vi "GEA2 Serial ICP Dryer SM.vi"(0 "ComPort":refnum<visa-resource-name>="COM1", 5 "Mode":T6=enum."Send WILT Startup CMDs", 7 "Xtra Command Data":u8[](array[numeric]) format="%02x", 9 "Dryer Status Serial Data In":T2, 11 "Error In":errorcluster, 13 "Command":T5 items=["CMD_Eval_Mode_Entry_CC1", "CMD_Eval_Mode_Entry_CC2", "CMD_Eval_Mode_Continue", "CMD_Send_DIAG_Info", "CMD_Enable_Debug_Log ", "CMD_Disable_Debug_Log ", "CMD_Send_Log_Data", "CMD_Stop", "RQST_Version"]) -> (4 "Dryer Status Serial Data Out":T2={"Color"=0, "Last Read Status"=enum."Err", "Command:Data"="", "Com Port"=0, "Time(S)"=0.0, "Err Count"=0}, 8 "DataReturned":u8[](array[numeric]) format="%.0x", 10 "WriteOK":bool, 14 "CRC Match":bool, 15 "Error Out":errorcluster)   [LabVIEW 2014]
uses:
  Type Definitions/GEA2 Serial Dryer Interface Ctrl.ctl
  Type Definitions/GEA2 Serial Dryer Commands.ctl
  Dryer Wilt/Type Definitions/WILT Dryer Com Port Info.ctl
  Dryer Wilt/Type Definitions/WILT Dryer Status Ctrl.ctl
  Type Definitions/Source Destination Control.ctl
  Type Definitions/GEA2 Serial Dryer Error Enumeration.ctl
  GEA2 Serial Globals Dryer.vi
  <vilib>/Instr/_visa.llb/VISA Configure Serial Port (Instr).vi
panel:
  in  "Source Destination 2":T1 {"Destination" format="%x"; "Source" format="%x"}
  in  "Source Destination":T1 {"Destination" format="%x"; "Source" format="%x"}
  in  "Total Bytes Read":i32
  in  "Tab Control 2":enum32{"Debug", "Serial Setup"}(tab)
  in  "Debug":bool
  out "State Array":string[](array[string])
  in  "Serial Timeout":u32=10
  out "Com:Data Buffer":string
  in  "Tab Control":T4(tab)
  in  "Exit":bool
  out "Com:Data":string
  out "Length":u8
  out "Source Read":u8 format="%.0x"
  out "Destination Read":u8 format="%.0x"
  out "Bytes At Port":u32=40
  out "Num Messages":dbl
  out "Read Pulse":dbl
  out "Partial Message":bool
  # "SubVI Commands"
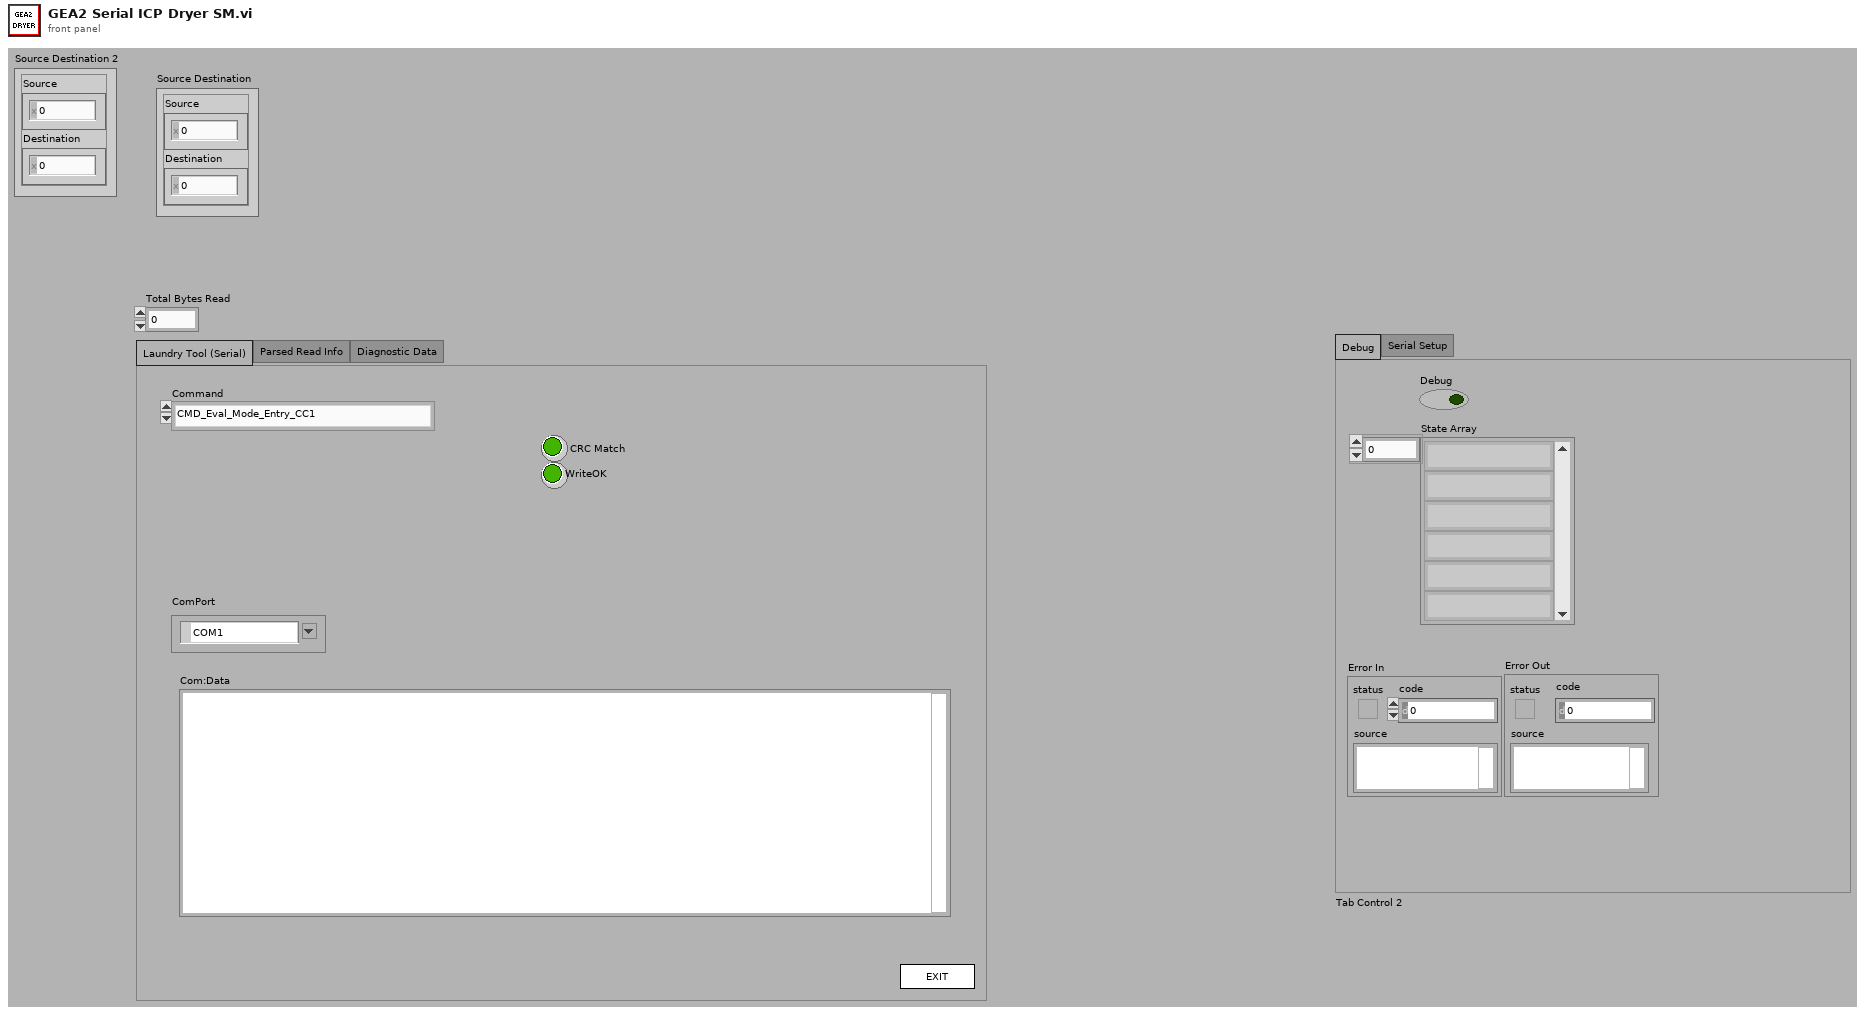
[diagram p1: front panel]
types:
  T1 = typedef "Source Destination Control.ctl" = cluster{"Source":u8, "Destination":u8}
  T2 = typedef "WILT Dryer Com Port Info.ctl" = cluster{"Color":u32, "Last Read Status":T3, "Command:Data":string, "Com Port":u8, "Time(S)":dbl, "Err Count":u32}
  T3 = typedef "WILT Dryer Status Ctrl.ctl" = enum16{"Cycle Not Started", "Cycle Running", "Paused", "Cycle Completed", "Eval Mode Entered", "Err", "Pause (No GEA2)"}
  T4 = enum32{"Laundry Tool (Serial)", "Parsed Read Info", "Diagnostic Data"}
  T5 = typedef "GEA2 Serial Dryer Commands.ctl" = u8
  T6 = typedef "GEA2 Serial Dryer Interface Ctrl.ctl" = enum16{"Init Com Port", "SendCMD", "ReadPort", "Close Port", "Simulate Diag Data", "Send WILT Startup CMDs", "Send Continue CMD", "Read Continuous"}
  T7 = enum32{"invalid app kind", "Development System", "Run Time System", "Student Edition", "Embedded LabVIEW", "Evaluation", "Custom"}
  T8 = enum32{"Invalid", "Standard", "Closed", "Hidden", "Minimized", "Maximized"}
  T9 = typedef "GEA2 Serial Dryer Error Enumeration.ctl" = enum16{"No Error", "GEA2 Send ACK Mismatch", "GEA2 STX", "GEA2 ETX", "GEA2 CRC Mismatch", "GEA2 ReadACK", "RTD In Range Error", "Fail Mean Tank Temp", "No Flow Config Data Found", "Failed Flow During Purge", "Temp During Purge", "Confirm IF Stop Fail", "Init Draw: TC_1 Out of Range", "Flow = 0 During Draw after 20s"}
  T10 = cluster{"Core":cluster{"Current VI Reference":refnum<vi>, "Close Panel on Exit?":bool}, "ComPort":refnum<visa-resource-name>, "ReadArray":u8[], "CRCArray":u8[], "Bytes Remaining":u8, "CRCRead":u8[], "CRC":bool, "Dryer Command":T5, "Error Out Flag":bool, "Bytes Data":u8[], "Dryer Status Serial Data In":T2, "Current Read Index":i32, "Total Bytes Read":i32, "Reset MSG Count":bool, "ACK":bool, "ReadCM1Flag":bool, "ReadCM2Flag":bool, "Reset Pulse":bool}
  T11 = cluster{"Current VI Reference":refnum<vi>, "Close Panel on Exit?":bool}
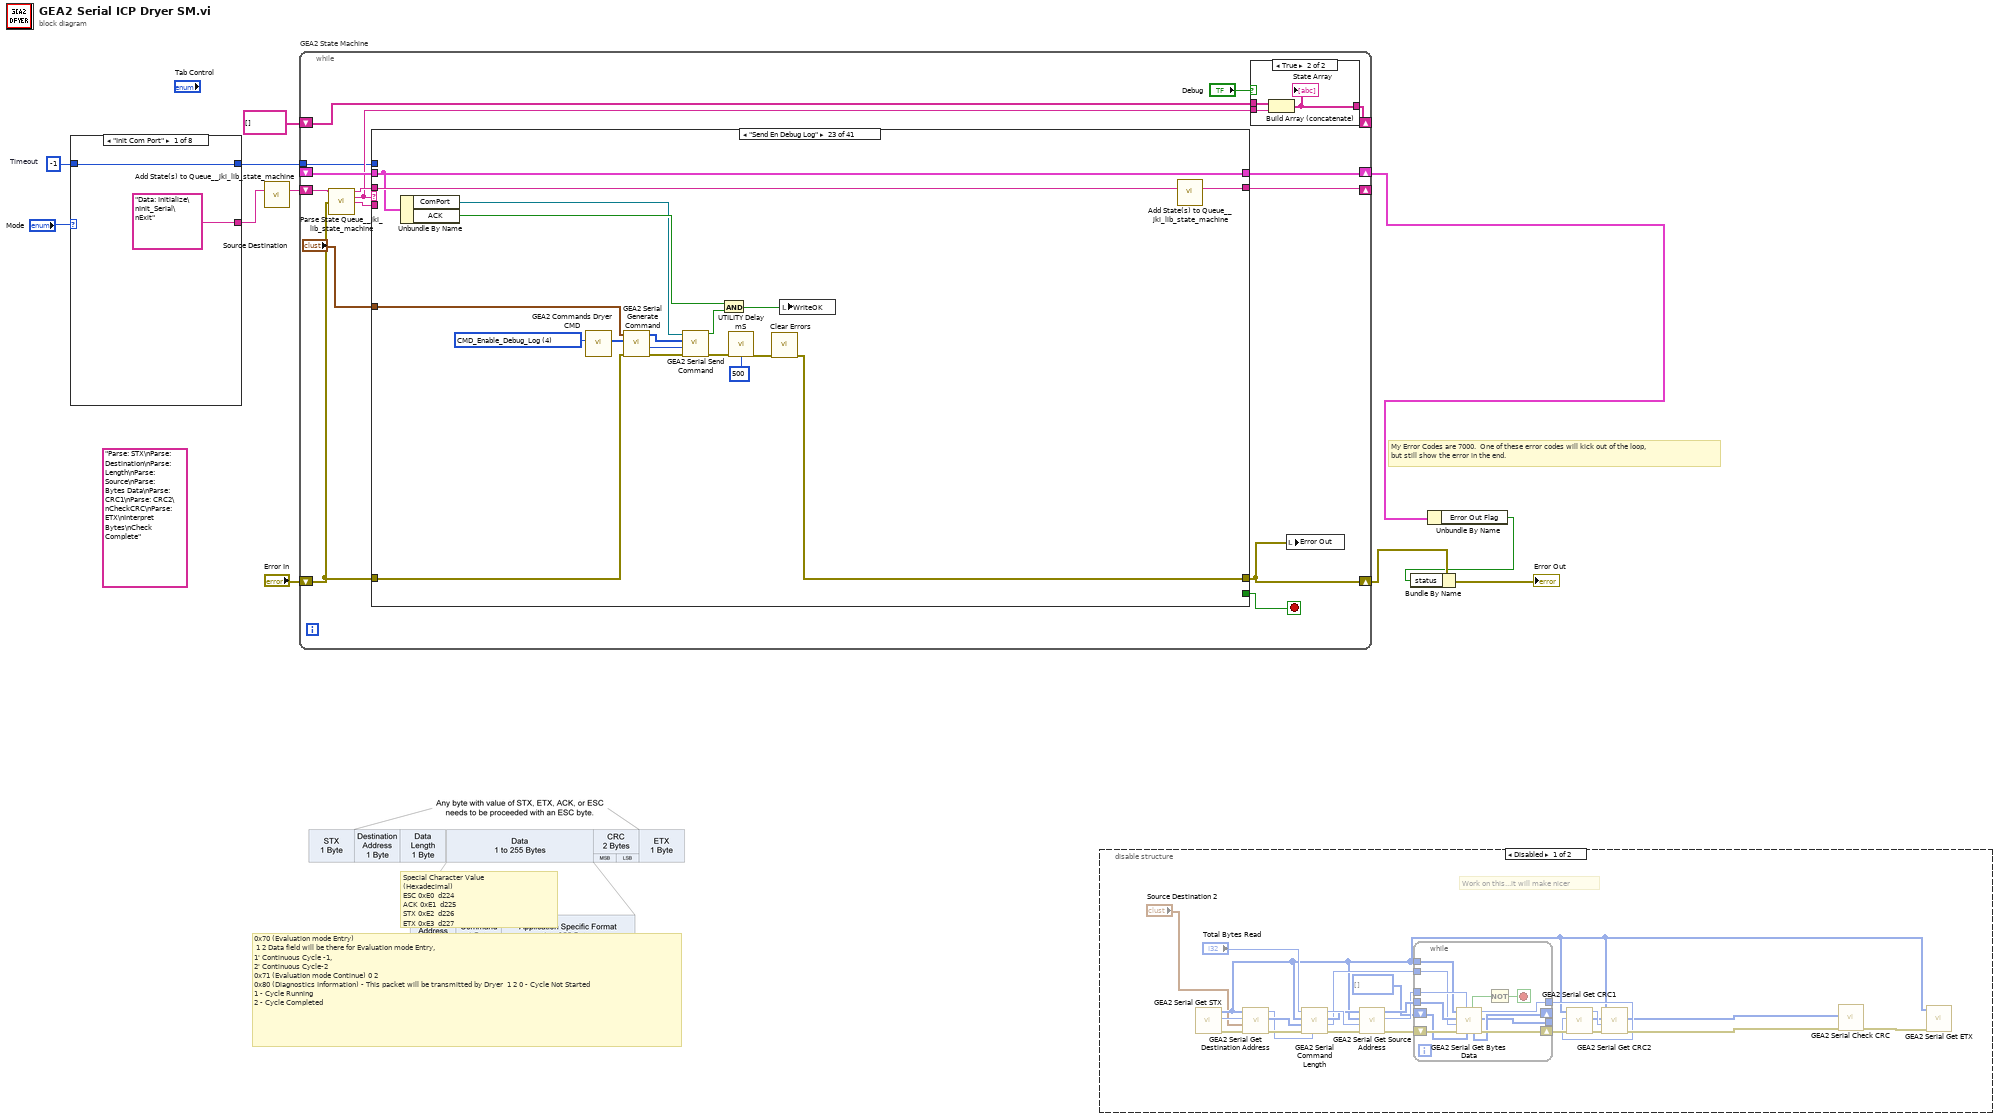
[diagram p0: block diagram]
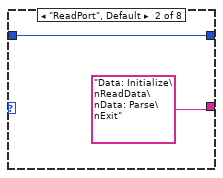
[diagram p3: hidden frame]
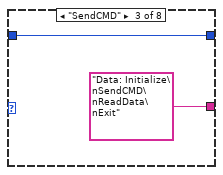
[diagram p4: hidden frame]
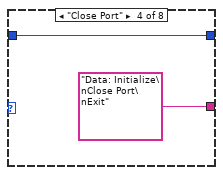
[diagram p5: hidden frame]
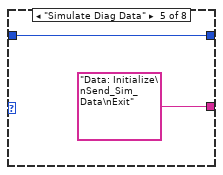
[diagram p6: hidden frame]
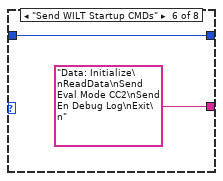
[diagram p7: hidden frame]
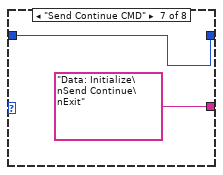
[diagram p8: hidden frame]
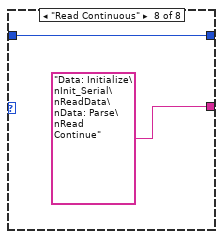
[diagram p9: hidden frame]
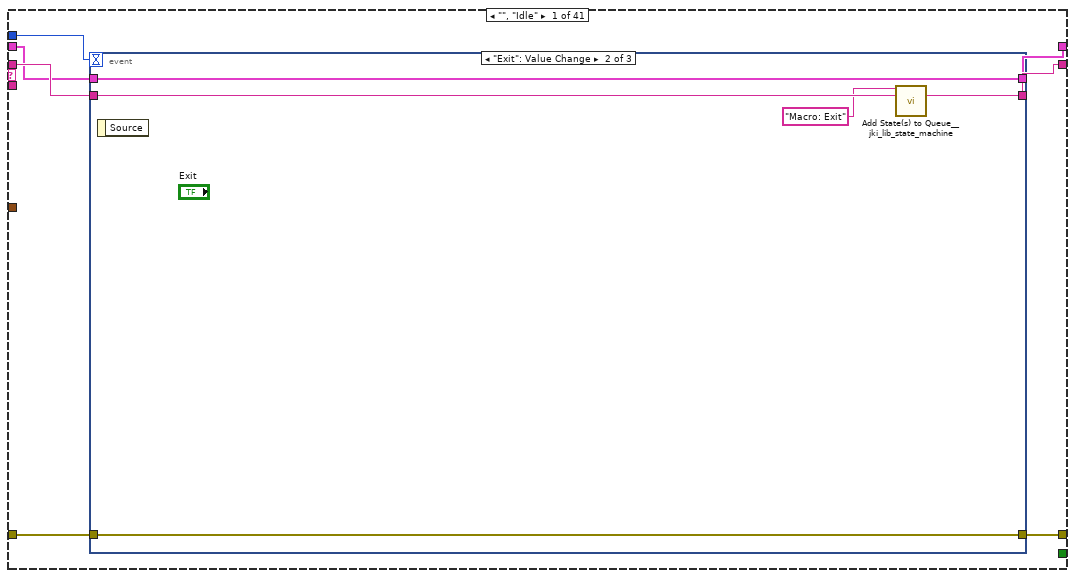
[diagram p11: hidden frame]
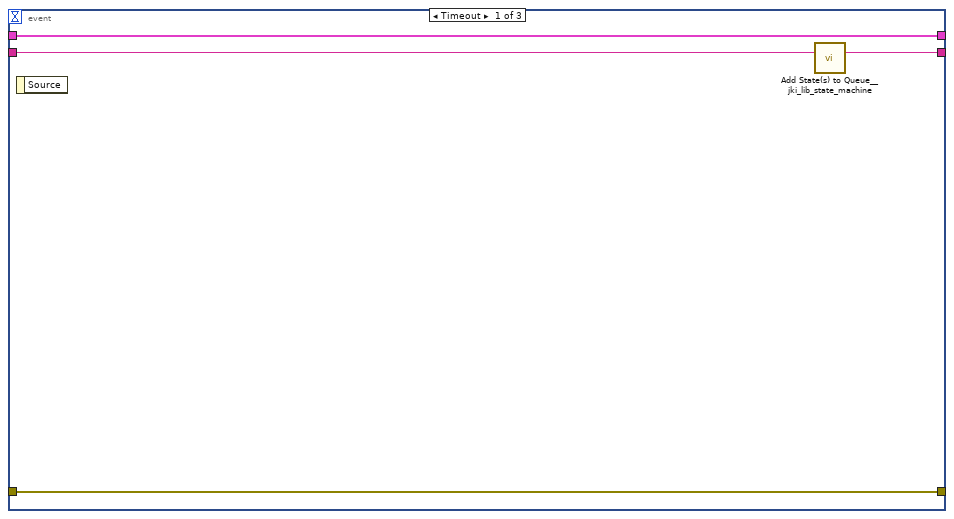
[diagram p12: hidden frame]
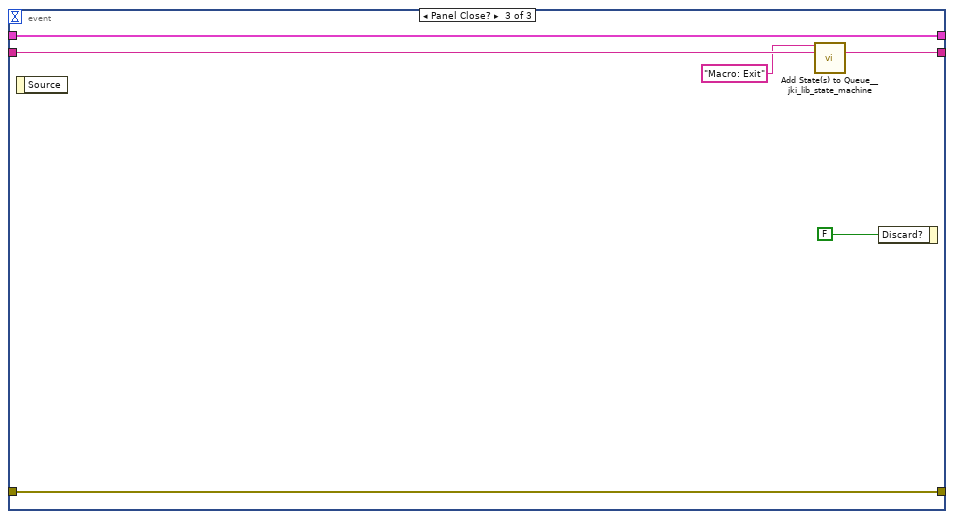
[diagram p13: hidden frame]
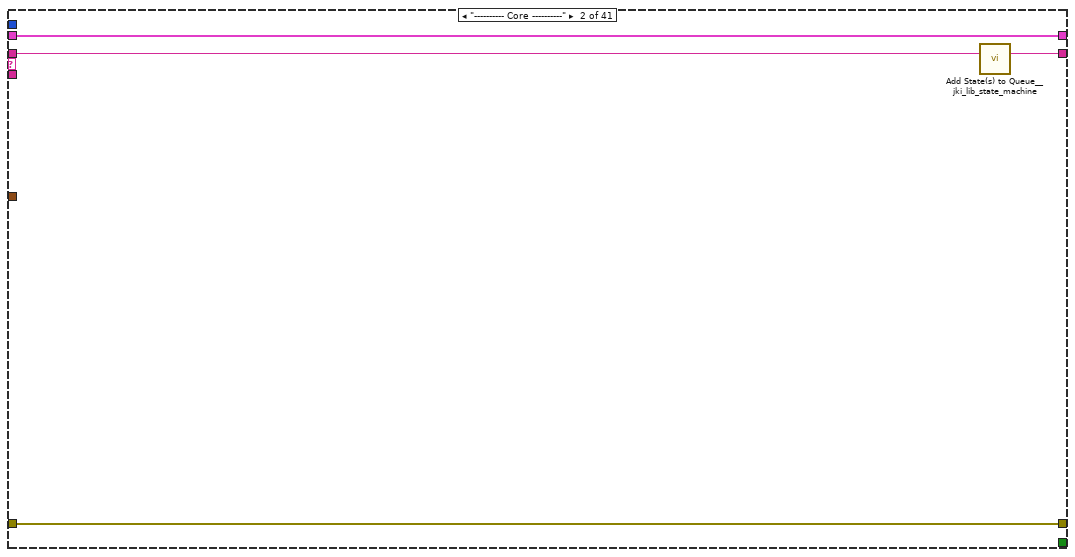
[diagram p14: hidden frame]
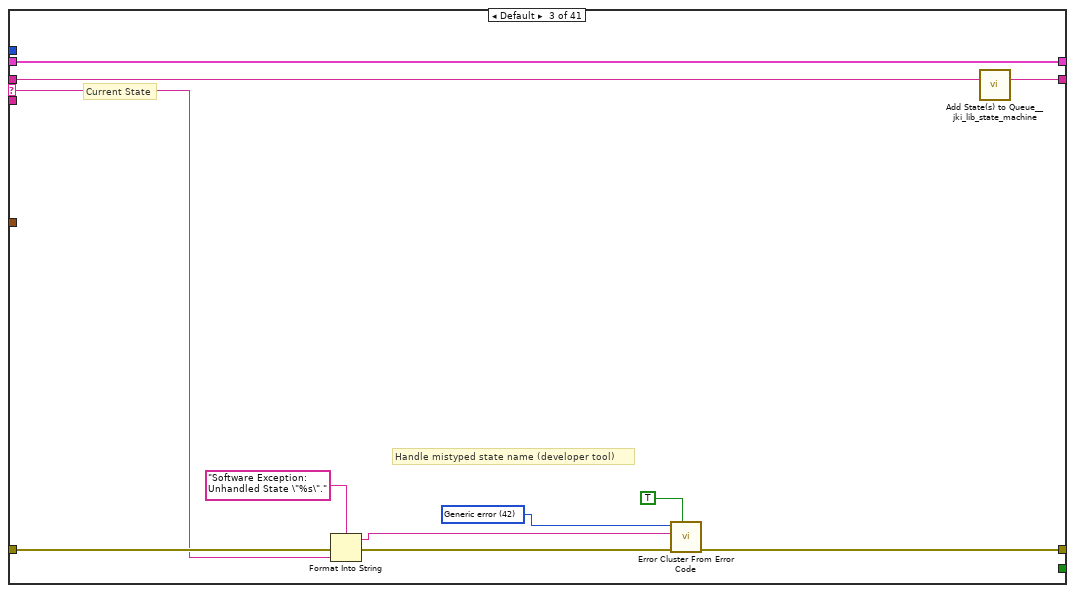
[diagram p15: hidden frame]
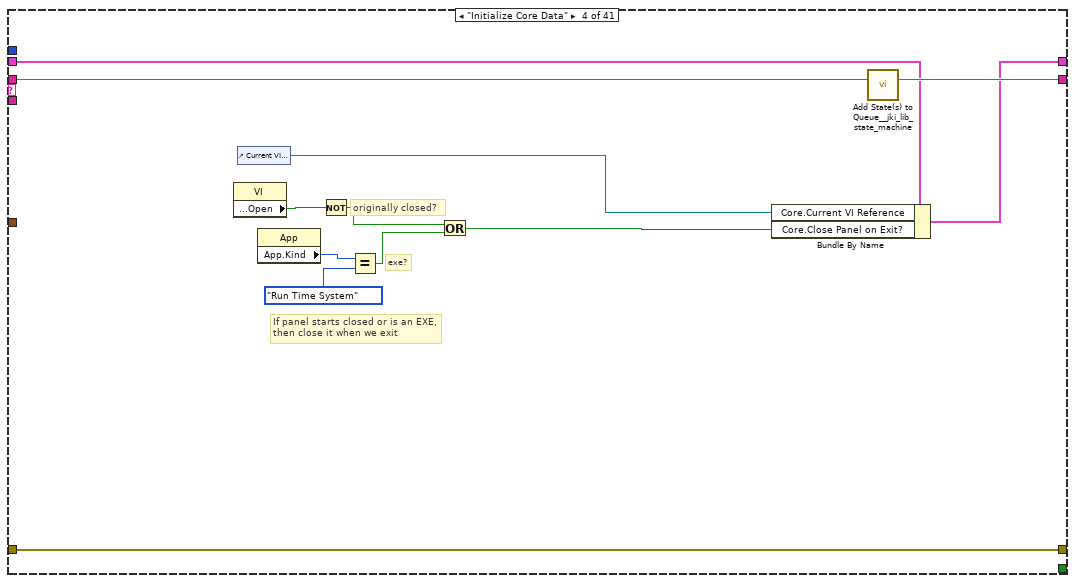
[diagram p16: hidden frame]
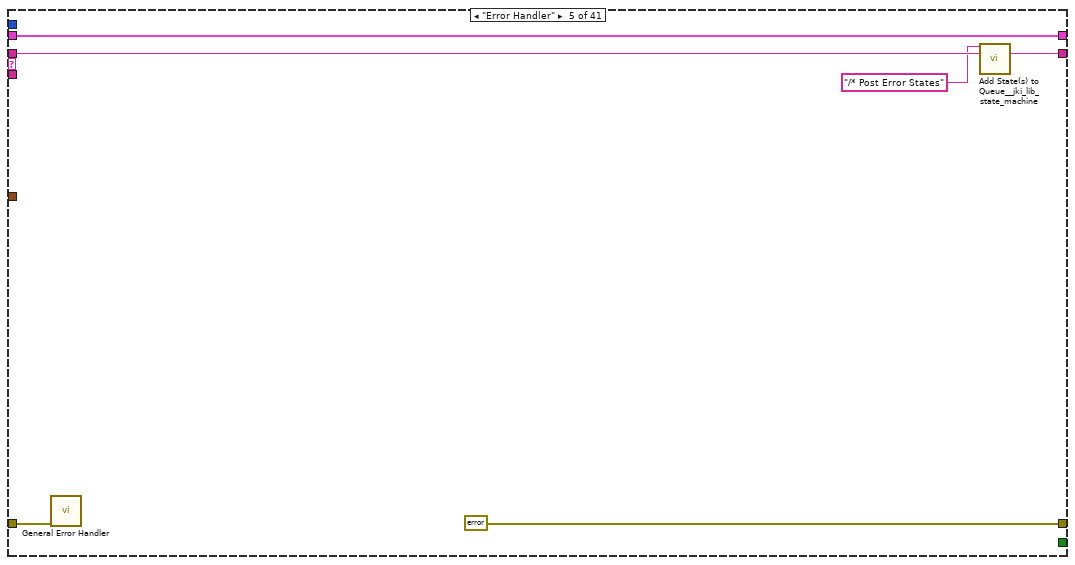
[diagram p17: hidden frame]
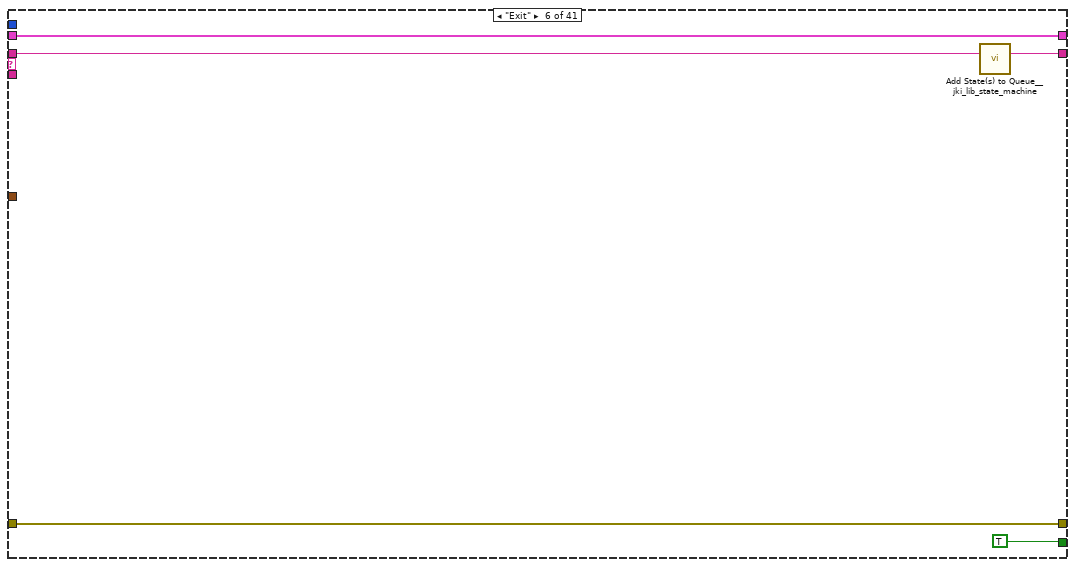
[diagram p18: hidden frame]
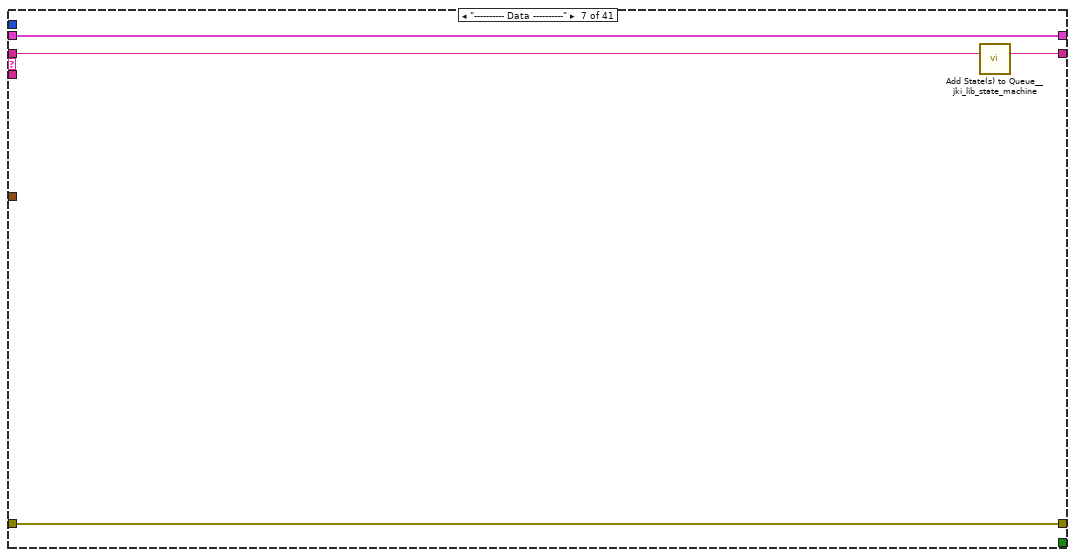
[diagram p19: hidden frame]
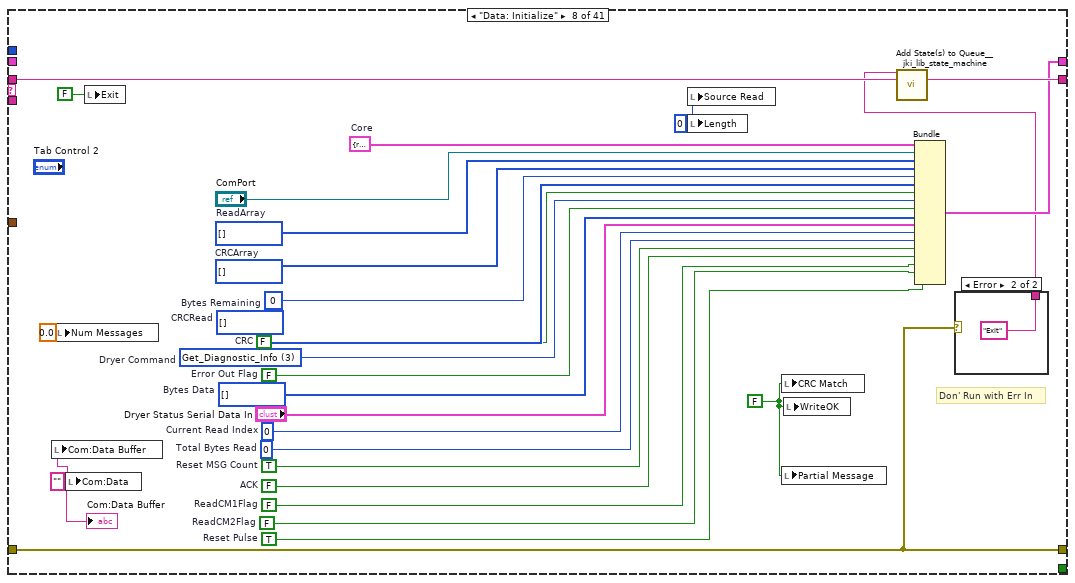
[diagram p20: hidden frame]
diagram:
  (unwired) "Parse: STX\nParse: Destination\nParse: Length\nParse: Source\nParse: Bytes Data\nParse: CRC1\nParse: CRC2\nCheckCRC\nParse: ETX\nInterpret Bytes\nCheck Complete" ("State(s) in Front (\"\")")
  w2 = -1  # Timeout
  # "0x70 (Evaluation mode Entry) \n\t1\t2\tData field will be there for Evaluation mode Entry, \n1' Continuous Cycle -1, \n2' Continuous Cycle-2\n0x71 (Evaluation mode Continue)\t0\t2\t\n0x80 (Diagnostics Information) - This packet will be transmitted by Dryer \t1\t2\t0 - Cycle Not Started\n1 - Cycle Running\n2 - Cycle Completed"
  # "My Error Codes are 7000.  One of these error codes will kick out of the loop,\nbut still show the error in the end."
  # "Special Character\tValue (Hexadecimal)\nESC\t0xE0  d224\nACK\t0xE1  d225\nSTX\t0xE2  d226\nETX\t0xE3  d227"
  n1 = case shown="\"Init Com Port\"" "Mode" {
    tunnel: ["Data: Initialize\nInit_Serial\nExit" "Data: Initialize\nReadData\nData: Parse\nExit" "Data: Initialize\nSendCMD\nReadData\nExit" "Data: Initialize\nClose Port\nExit" "Data: Initialize\nSend_Sim_Data\nExit" "Data: Initialize\nReadData\nSend Eval Mode CC2\nSend En Debug Log\nExit\n" "Data: Initialize\nSend Continue\nExit" "Data: Initialize\nInit_Serial\nReadData\nData: Parse\nRead Continue"] -> w1
    tunnel: [w12 w14 w16 w18 w20 w22 w24 w27] -> w3
    tunnel: w2 -> [w12 w14 w16 w18 w20 w22 w24 w27]
    frame "Init Com Port" {
    }
    frame "ReadPort", Default {
    }
    frame "SendCMD" {
    }
    frame "Close Port" {
    }
    frame "Simulate Diag Data" {
    }
    frame "Send WILT Startup CMDs" {
    }
    frame "Send Continue CMD" {
    }
    frame "Read Continuous" {
    }
  }
  n2 = call <vilib>:"Add State(s) to Queue__jki_lib_state_machine.vi"("State(s) in (\"\")"=w1) -> ("States Out"=w11:string)  [unwired: 14 in]
  n3 = while "GEA2 State Machine" {
    shift-right: [w38] -> w6
    shift-left: _ -> [w37]
    shift-right: [w34] -> w9
    shift-left: "Error In" -> [w36]
    shift-right: [w35] -> _
    shift-left: w11 -> [w40]
    shift-right: [w31] -> _
    shift-left: string[] [] -> [w33]
    tunnel: w3 -> [w30]
    stop <- w39 stop-if-true
    n4 = call <vilib>:"Parse State Queue__jki_lib_state_machine.vi"("State Queue"=w40, "Error In (no error)"=w36) -> ("Remaining States"=w42:string, "Current State"=w32:string, "Arguments"=w41:string)  [unwired: 11 in]
    n5 = case shown="\"Send En Debug Log\"" w32 {
      selector: w32 -> [_ _ w73 _ _ _ _ _ _ _ _ _ _ _ _ _ _ _ _ _ _ _ _ _ _ _ _ _ _ _ _ _ _ _ _ _ _ _ _ _ _]
      tunnel: w42 -> [w53 w72 w77 w95 w101 w102 w110 w138 w145 w149 w153 w159 w170 w196 w201 w211 w215 w241 w252 w270 w287 w302 w320 w334 w346 w363 w367 w376 w396 w415 w423 w449 w466 w478 w489 w498 w510 w524 w534 w548 w574]
      tunnel: w41 -> [_ _ _ _ _ _ _ _ _ _ _ w154 w164 _ _ _ _ _ _ _ _ _ _ _ _ _ _ _ _ _ _ _ _ _ _ _ _ _ _ _ _]
      tunnel: w37 -> [w51 w69 w75 w86 w97 w104 w107 _ w142 w146 w151 w157 w166 w193 w198 w208 w212 w238 w249 w262 w284 w299 w317 w330 w344 w360 w364 w370 w394 w413 w431 w447 w464 w476 w487 w494 w508 w519 w529 w537 w555]
      tunnel: [w50 w70 w79 w92 errorcluster {"status"=FALSE, "code"=0, "source"=""} ("error out") w105 w108 w124 w140 w147 w150 w155 w167 w194 w199 w209 w213 w239 w250 w264 w282 w297 w312 w321 w335 w347 w365 w374 w392 w404 w416 w438 w451 w469 w479 w492 w505 w520 w532 w546 w572] -> w34
      tunnel: w36 -> [w49 w70 w78 w92 w99 w105 w108 w124 w143 w147 w150 w156 w168 w194 w199 w209 w213 w225 w247 w255 w279 w296 w311 w331 w338 w354 w365 w374 w386 w405 w417 w439 w452 w470 w480 w496 w500 w522 w532 w546 w572]
      tunnel: [w52 w71 w76 w94 w100 w106 w109 w137 w144 w148 w152 w158 w169 w195 w200 w210 w214 w240 w251 w269 w286 w301 w319 w333 w345 w362 w366 w375 w395 w414 w432 w448 w465 w477 w488 w497 w509 w523 w533 w547 w573] -> w35
      tunnel: [_ _ _ _ _ TRUE _ _ _ _ _ _ _ _ _ _ _ _ _ _ _ _ _ _ _ _ _ _ _ _ _ _ _ _ _ _ _ _ _ _ _] -> w39
      tunnel: [w48 w69 w75 w93 w97 w104 w107 w136 w142 w146 w151 w157 w166 w193 w198 w208 w212 w237 w249 w262 w283 w299 w317 w330 w344 w356 w364 w369 w393 w412 w430 w446 w463 w475 w486 w493 w507 w519 w528 w536 w571] -> w38
      tunnel: w30 -> [w47 _ _ _ _ _ _ _ _ _ _ _ _ _ _ _ _ _ _ _ _ _ _ _ _ _ _ _ _ _ _ _ _ _ _ _ _ _ _ _ _]
      tunnel: "Source Destination" -> [_ _ _ _ _ _ _ _ _ _ _ _ _ _ _ _ _ _ _ w253 w281 w293 w310 w329 w343 _ _ _ _ _ _ w441 _ _ _ _ _ _ _ _ _]
      frame "", "Idle" {
        n6 = event shown="[1] \"Exit\": Value Change" {
          selector: _ -> [_ _ _]
          dyn-events: _ -> [_ _ _]
          timeout: w47 -> [_ _ _]
          tunnel: w53 -> [w57 w62 w68]
          tunnel: [w56 w61 w67] -> w52
          tunnel: w51 -> [w54 w59 w65]
          tunnel: [w55 w60 w66] -> w50
          tunnel: w49 -> [w55 w60 w66]
          tunnel: [w54 w59 w65] -> w48
          event Timeout {
            n7 = event-data() -> ()  [unwired: 1 in, 1 out]
            n8 = call <vilib>:"Add State(s) to Queue__jki_lib_state_machine.vi"("State(s) in (\"\")"=w57) -> ("States Out"=w56:string)  [unwired: 14 in]
          }
          event "Exit": Value Change {
            n9 = event-data() -> ()  [unwired: 1 in, 1 out]
            n10 = call <vilib>:"Add State(s) to Queue__jki_lib_state_machine.vi"("State(s) in Front (\"\")"="Macro: Exit", "State(s) in (\"\")"=w62) -> ("States Out"=w61:string)  [unwired: 13 in]
          }
          event Panel Close? {
            n11 = event-data() -> ()  [unwired: 1 in, 1 out]
            n12 = call <vilib>:"Add State(s) to Queue__jki_lib_state_machine.vi"("State(s) in Front (\"\")"="Macro: Exit", "State(s) in (\"\")"=w68) -> ("States Out"=w67:string)  [unwired: 13 in]
            n13 = event-data("Discard?"=FALSE) -> ()  [unwired: 1 in, 1 out]
          }
        }
      }
      frame "---------- Core ----------" {
        n14 = call <vilib>:"Add State(s) to Queue__jki_lib_state_machine.vi"("State(s) in (\"\")"=w72) -> ("States Out"=w71:string)  [unwired: 14 in]
      }
      frame Default {
        w82 = 42 items=["No error", "Argument error", "Memory is full", "Out of zone", "End of file", "File already open", "Generic file I/O error", "File not found", "File permission error", "Disk is full", "Duplicate path", "Too many files open", "System feature not enabled", "Resource file not found", "Cannot add resource", "Resource not found", "Image not found", "Image memory error", "Pen does not exist", "Config type invalid", "Config token not found", "Config parse error", "Config memory error", "Bad external code format", "Bad external code offset", "External code not present", "Null window", "Destroy window error", "Null menu", "Print aborted", "Bad print record", "Print driver error", "Windows error during printing", "Memory error during printing", "Print dialog error", "Generic print error", "Invalid device refnum", "Device not found", "Device parameter error", "Device unit error", "Cannot open device", "Device call aborted", "Generic error", "Cancelled by user", "Object ID too low", "Object ID too high", "Object not in heap", "Unknown heap", "Unknown object (invalid DefProc)", "Unknown object (DefProc not in table)", "Message out of range", "Invalid (null) method", "Unknown message", "Manager call not supported", "Bad address", "Network operation in progress", "Network operation timed out", "Connection is busy", "Network attribute not supported", "Network error", "Address in use", "System out of memory", "Connection aborted", "Connection refused", "Not connected", "Already connected", "Connection closed", "Initialization error (interapplication manager)", "Bad occurrence", "Wait on unbound occurrence handler", "Occurrence queue overflow", "Datalog type conflict", "Unused", "Unrecognized type (interapplication manager)", "Memory corrupt", "Failed to make temporary DLL", "Old CIN version", "Drag socket not found", "Failed to load drop-object", "Failed to register OLE object", "Failed to release OLE object", "Format specifier type mismatch", "Unknown format specifier", "Too few format specifiers", "Too many format specifiers", "Scan failed", "Newer CIN version", "Error converting to variant", "Runtime menu error", "Password tampered", "Variant attribute not found", "Incompatible variant data type", "Event data is not available", "Event Store is not present", "Occurrence is not found", "Event Queue is not created", "Event info is not available", "Refnum passed is NULL", "Error retrieving Class GUID", "Error retrieving CoClass GUID", "Error retrieving TypeLib GUID.", "Bad built application magic bytes.", "Specific driver is different from the specific driver associated with the Logical Name.", "There is no session opened to the class driver.", "Max Error", "MAX - Error with config objects", "MAX - Error loading configuration", "MAX - Group not supported"]
        # "Current State"
        # "Handle mistyped state name (developer tool)"
        n15 = Format Into String(format string="Software Exception: Unhandled State \"%s\"." ("message"), error in=w78, w73) -> (resulting string=w81:string, error out=w80:errorcluster)  [unwired: 1 in]
        n16 = call <vilib>:"Error Cluster From Error Code.vi"("show call chain? (False)"=TRUE, "error in (no error)"=w80, "error message (\"\")"=w81, "error code (0)"=w82) -> ("error out"=w79:errorcluster)  [unwired: 5 in]
        n17 = call <vilib>:"Add State(s) to Queue__jki_lib_state_machine.vi"("State(s) in (\"\")"=w77) -> ("States Out"=w76:string)  [unwired: 14 in]
      }
      frame "Initialize Core Data" {
        # "originally closed?"
        # "exe?"
        # "If panel starts closed or is an EXE, then close it when we exit"
        n18 = property class="VI"() -> ("Front Panel.Open"=w91:bool)  [unwired: 2 in, 2 out]
        n19 = control-ref of="Current VI Reference"() -> (w84:refnum<vi>)
        n20 = property class="App"() -> ("App.Kind"=w90:T7)  [unwired: 2 in, 2 out]
        n21 = Not(x=w91) -> (.not. x?=w88:bool)
        n22 = Equal?(x=w90, y=T7."Run Time System" ("Application:Kind")) -> (x = y?=w87:bool)
        n23 = Or(x=w88, y=w87) -> (x .or. y?=w85:bool)
        n24 = Bundle By Name(cluster=w86, "Core.Current VI Reference"=w84, "Core.Close Panel on Exit?"=w85) -> (w93:T10)
        n25 = call <vilib>:"Add State(s) to Queue__jki_lib_state_machine.vi"("State(s) in (\"\")"=w95) -> ("States Out"=w94:string)  [unwired: 14 in]
      }
      frame "Error Handler" {
        n26 = call <vilib>:"General Error Handler.vi"("error in (no error)"=w99) -> ()  [unwired: 10 in, 5 out]
        n27 = call <vilib>:"Add State(s) to Queue__jki_lib_state_machine.vi"("State(s) in Front (\"\")"="/* Post Error States", "State(s) in (\"\")"=w101) -> ("States Out"=w100:string)  [unwired: 13 in]
      }
      frame "Exit" {
        n28 = call <vilib>:"Add State(s) to Queue__jki_lib_state_machine.vi"("State(s) in (\"\")"=w102) -> ("States Out"=w106:string)  [unwired: 14 in]
      }
      frame "---------- Data ----------" {
        n29 = call <vilib>:"Add State(s) to Queue__jki_lib_state_machine.vi"("State(s) in (\"\")"=w110) -> ("States Out"=w109:string)  [unwired: 14 in]
      }
      frame "Data: Initialize" {
        w112 = TRUE  # Reset Pulse
        w115 = FALSE  # ReadCM2Flag
        w116 = FALSE  # ReadCM1Flag
        w113 = "" ("Com:Data")
        w117 = FALSE  # ACK
        w118 = TRUE  # Reset MSG Count
        w119 = 0  # Total Bytes Read
        w120 = 0  # Current Read Index
        w125 = u8 0 ("Length")
        w126 = T5 3 items=["Eval_Mode_Entry_CC1", "Eval_Mode_Entry_CC2", "Eval_Mode_Continue", "Get_Diagnostic_Info"]  # Dryer Command
        w127 = u8[] []  # Bytes Data
        w128 = T11 {"Current VI Reference"=refnum, "Close Panel on Exit?"=FALSE}  # Core
        w114 = FALSE ("CRC Match")
        w129 = FALSE  # Error Out Flag
        w130 = FALSE  # CRC
        w131 = u8[] []  # CRCRead
        w132 = u8 0  # Bytes Remaining
        w133 = u8[] []  # CRCArray
        w134 = u8[] []  # ReadArray
        # "Don' Run with Err In"
        n30 = local write "Com:Data Buffer"(w113) -> ()
        n31 = local write "Num Messages"(0.0 ("Num Messages")) -> ()
        n32 = local write "Com:Data"(w113) -> ()
        n33 = local write "Exit"(FALSE ("Start Pressed")) -> ()
        n34 = local write "Source Read"(w125) -> ()
        n35 = local write "Length"(w125) -> ()
        n36 = local write "CRC Match"(w114) -> ()
        n37 = local write "Partial Message"(w114) -> ()
        n38 = local write "WriteOK"(w114) -> ()
        n39 = Bundle("Core"=w128, "ComPort"="ComPort", "ReadArray"=w134, "CRCArray"=w133, "Bytes Remaining"=w132, "CRCRead"=w131, "CRC"=w130, "Dryer Command"=w126, "Error Out Flag"=w129, "Bytes Data"=w127, "Dryer Status Serial Data In"="Dryer Status Serial Data In", "Current Read Index"=w120, "Total Bytes Read"=w119, "Reset MSG Count"=w118, "ACK"=w117, "ReadCM1Flag"=w116, "ReadCM2Flag"=w115, "Reset Pulse"=w112) -> (w136:T10)  [unwired: 1 in]
        n40 = case shown="Error" w124 {
          tunnel: [_ "Exit"] -> w123
          frame No Error {
          }
          frame Error {
          }
        }
        n41 = call <vilib>:"Add State(s) to Queue__jki_lib_state_machine.vi"("State(s) in Front (\"\")"=w123, "State(s) in (\"\")"=w138) -> ("States Out"=w137:string)  [unwired: 13 in]
        "Com:Data Buffer" <- w113
      }
      frame "Data: Cleanup" {
        n42 = Unbundle By Name(w142) -> ("Core.Current VI Reference"=w141:refnum<vi>)
        n43 = Close Reference(reference=w141, error in (no error)=w143) -> (error out=w140:errorcluster)
        n44 = call <vilib>:"Add State(s) to Queue__jki_lib_state_machine.vi"("State(s) in (\"\")"=w145) -> ("States Out"=w144:string)  [unwired: 14 in]
      }
      frame "---------- UI ----------" {
        n45 = call <vilib>:"Add State(s) to Queue__jki_lib_state_machine.vi"("State(s) in (\"\")"=w149) -> ("States Out"=w148:string)  [unwired: 14 in]
      }
      frame "UI: Initialize" {
        n46 = call <vilib>:"Add State(s) to Queue__jki_lib_state_machine.vi"("State(s) in (\"\")"=w153) -> ("States Out"=w152:string)  [unwired: 14 in]
      }
      frame "UI: Cursor Set" {
        # "Argument"
        n47 = case shown="\"Idle\", Default" w154 {
          tunnel: w156 -> [w161 w163]
          tunnel: [w160 w162] -> w155
          frame "Idle", Default {
            n48 = call <vilib>:"Unset Busy.vi"("error in (no error)"=w161) -> ("error out"=w160:errorcluster)  [unwired: 10 in]
          }
          frame "Busy" {
            n49 = call <vilib>:"Set Busy.vi"("error in (no error)"=w163) -> ("error out"=w162:errorcluster)  [unwired: 9 in, 1 out]
          }
        }
        n50 = call <vilib>:"Add State(s) to Queue__jki_lib_state_machine.vi"("State(s) in (\"\")"=w159) -> ("States Out"=w158:string)  [unwired: 14 in]
      }
      frame "UI: Front Panel State" {
        # "Argument"
        n51 = Unbundle By Name(w166) -> ("Core.Current VI Reference"=w165:refnum<vi>)
        n52 = case shown="\"Close\"" w164 {
          tunnel: w168 -> [w174 w187]
          tunnel: [w176 w188] -> w167
          tunnel: w165 -> [w175 w185]
          frame "Open", Default {
            n53 = property class="VI"(reference=w175, error in=w174) -> (reference out=w172:refnum<vi>, error out=w173:errorcluster, "Front Panel.Open"=w171:bool)
            n54 = case shown="False" w171 {
              tunnel: [w179 w182] -> w176
              tunnel: w173 -> [w178 w182]
              tunnel: w172 -> [w177 _]
              frame False {
                n55 = invoke class="VI" method="FP.Open"(reference=w177, error in=w178, "Activate"=TRUE, "State"=T8."Standard") -> (error out=w179:errorcluster)  [unwired: 1 in, 4 out]
              }
              frame True {
              }
            }
          }
          frame "Close" {
            n56 = property class="VI"(reference=w185, error in=w187) -> (reference out=w184:refnum<vi>, error out=w186:errorcluster, "Front Panel.Open"=w183:bool)
            n57 = case shown="True" w183 {
              tunnel: [w189 w192] -> w188
              tunnel: w186 -> [w189 w191]
              tunnel: w184 -> [_ w190]
              frame False {
              }
              frame True {
                n58 = invoke class="VI" method="FP.Close"(reference=w190, error in=w191) -> (error out=w192:errorcluster)  [unwired: 1 in, 2 out]
              }
            }
          }
        }
        n59 = call <vilib>:"Add State(s) to Queue__jki_lib_state_machine.vi"("State(s) in (\"\")"=w170) -> ("States Out"=w169:string)  [unwired: 14 in]
      }
      frame "---------- Macro ----------" {
        n60 = call <vilib>:"Add State(s) to Queue__jki_lib_state_machine.vi"("State(s) in (\"\")"=w196) -> ("States Out"=w195:string)  [unwired: 14 in]
      }
      frame "Macro: Initialize" {
        w197 = "Data: Initialize\nInitialize Core Data\nUI: Initialize\nUI: Front Panel State >> Open\nInit_Serial"  # Data: Initialize Initialize Core Data UI: Initialize UI: Front Panel State >> Open Init_Serial
        n61 = call <vilib>:"Add State(s) to Queue__jki_lib_state_machine.vi"("State(s) in Front (\"\")"=w197, "State(s) in (\"\")"=w201) -> ("States Out"=w200:string)  [unwired: 13 in]
      }
      frame "Macro: Exit" {
        n62 = Unbundle By Name(w208) -> ("Core.Close Panel on Exit?"=w202:bool)
        n63 = Select(t="UI: Front Panel State >> Close", s=w202, f="") -> (s? t:f=w204:string)
        n64 = call <vilib>:"Add State(s) to Queue__jki_lib_state_machine.vi"("State(s) in (\"\")"=w204, "State(s) at Back (\"\")"="Data: Cleanup\nExit") -> ("States Out"=w207:string)  [unwired: 13 in]
        n65 = call <vilib>:"Add State(s) to Queue__jki_lib_state_machine.vi"("State(s) in Front (\"\")"=w207, "State(s) in (\"\")"=w211) -> ("States Out"=w210:string)  [unwired: 13 in]
      }
      frame "---------- New Category ----------" {
        n66 = call <vilib>:"Add State(s) to Queue__jki_lib_state_machine.vi"("State(s) in (\"\")"=w215) -> ("States Out"=w214:string)  [unwired: 14 in]
      }
      frame "Init_Serial" {
        w232 = u16 0 items=["None", "XON/XOFF", "RTS/CTS", "XON/XOFF & RTS/CTS", "DTR/DSR", "XON/XOFF & DTR/DSR"] ("flow control (0:none)")
        w231 = u16 10 items=["1.0"=10, "1.5"=15, "2.0"=20] ("stop bits (10: 1 bit)")
        # "skip error handle routine"
        # "Assumes that if the serial port is 19200, then it is all ok."
        n67 = Unbundle By Name(w238) -> ("ComPort"=w219:refnum<visa-resource-name>)
        n68 = call "UTILITY Com Chan Type Conversion.vi"("Com Chan In"=w219) -> ("Com Channel #"=w218:u8)  [unwired: 11 in, 3 out]
        n69 = global read "GEA2 Serial Globals Dryer.vi" "No Com Color"() -> (w224:u32)
        n70 = Bundle By Name(cluster=T2 {"Color"=0, "Last Read Status"=enum."Err", "Command:Data"="", "Com Port"=0, "Time(S)"=0.0, "Err Count"=0} ("Dryer Status Serial Data Out"), "Color"=w224, "Last Read Status"=WILT_Dryer_Status_Ctrl."Err", "Command:Data"="", "Com Port"=w218, "Time(S)"=0.0, "Err Count"=u32 0) -> (w217:T2)
        n71 = local write "Dryer Status Serial Data Out"(w217) -> ()
        n72 = call-poly "VISA Configure Serial Port"("VISA resource name"=w219, "timeout (10sec)"="Serial Timeout", "Enable Termination\nChar (T)"=FALSE ("Enable Termination\nChar (T)"), "baud rate (9600)"=u32 19200, "data bits (8)"=u16 8, "parity (0:none)"=enum16{"None", "Odd", "Even", "Mark", "Space"}."None", "error in (no error)"=w225, "stop bits (10: 1 bit)"=w231, "flow control (0:none)"=w232) -> ("VISA resource name out"=w234:refnum<visa-resource-name>, "error out"=w235:errorcluster)  [unwired: 5 in]
        n73 = Equal To 0?(x="Serial Timeout") -> (x = 0?=w227:bool)
        n74 = case shown="True" w227 {
          tunnel: w235 -> [w242 w245]
          tunnel: w234 -> [_ w244]
          tunnel: [w242 w243] -> w239
          frame False {
          }
          frame True {
            n75 = VISA Flush I/O Buffer(VISA resource name=w244, error in (no error)=w245) -> (error out=w243:errorcluster)  [unwired: 1 in, 1 out]
          }
        }
        n76 = Bundle By Name(cluster=w238, "ComPort"=w234) -> (w237:T10)
        n77 = call <vilib>:"Add State(s) to Queue__jki_lib_state_machine.vi"("State(s) in Front (\"\")"="" ("State(s) in Front (\"\")"), "State(s) in (\"\")"=w241) -> ("States Out"=w240:string)  [unwired: 13 in]
      }
      frame "Close Port" {
        n78 = Unbundle By Name(w249) -> ("ComPort"=w246:refnum<visa-resource-name>)
        n79 = VISA Close(VISA resource name=w246, error in (no error)=w247) -> (error out=w250:errorcluster)
        n80 = call <vilib>:"Add State(s) to Queue__jki_lib_state_machine.vi"("State(s) in Front (\"\")"="" ("State(s) in Front (\"\")"), "State(s) in (\"\")"=w252) -> ("States Out"=w251:string)  [unwired: 13 in]
      }
      frame "SendCMD" {
        n81 = Unbundle By Name(w262) -> ("ComPort"=w268:refnum<visa-resource-name>)
        n82 = call "GEA2 Commands Dryer CMD.vi"("Dryer Cmd"="Command") -> ("CMD Array"=w267:u8[])  [unwired: 10 in]
        n83 = call "GEA2 Serial Generate Command.vi"("Error In"=w255, "Xtra Command Data"="Xtra Command Data", "CMD Array"=w267, "Source Destination"=w253) -> ("Error Out"=w254:errorcluster, "Byte Count"=w257:u32, "Message Out"=w258:u8[])  [unwired: 5 in]
        n84 = call "GEA2 Serial Send Command.vi"("error in (no error)"=w254, "Byte Count"=w257, "Message Out"=w258, "VISA Refnum in"=w268) -> ("error out"=w265:errorcluster, "WriteOK"=→"WriteOK":bool)  [unwired: 6 in]
        n85 = call "UTILITY Delay mS.vi"("Error In"=w265, "milliseconds to wait"=u32 10) -> ("Error Out"=w264:errorcluster)  [unwired: 13 in]
        n86 = call "GEA2 Serial Dryer Command Needs Read.vi"("Command 2"="Command") -> ("RQST"=w260:bool)  [unwired: 13 in, 1 out]
        n87 = case shown="False" w260 {
          tunnel: ["" "ReadData\nData: Parse"] -> w259
          frame False {
          }
          frame True {
          }
        }
        n88 = call <vilib>:"Add State(s) to Queue__jki_lib_state_machine.vi"("State(s) in Front (\"\")"=w259, "State(s) in (\"\")"=w270) -> ("States Out"=w269:string)  [unwired: 13 in]
      }
      frame "Send Eval Mode CC2" {
        w285 = T5 1 items=["CMD_Eval_Mode_Entry_CC1", "CMD_Eval_Mode_Entry_CC2", "CMD_Eval_Mode_Continue", "CMD_Send_DIAG_Info", "CMD_Enable_Debug_Log ", "CMD_Disable_Debug_Log ", "CMD_Send_Log_Data"] ("Command 2")
        n89 = Unbundle By Name(w284) -> ("ComPort"=w278:refnum<visa-resource-name>)
        n90 = call "GEA2 Commands Dryer CMD.vi"("Dryer Cmd"=w285) -> ("CMD Array"=w280:u8[])  [unwired: 10 in]
        n91 = call "GEA2 Serial Generate Command.vi"("Error In"=w279, "CMD Array"=w280, "Source Destination"=w281) -> ("Error Out"=w277:errorcluster, "Byte Count"=w275:u32, "Message Out"=w276:u8[])  [unwired: 6 in]
        n92 = call "GEA2 Serial Send Command.vi"("error in (no error)"=w277, "Byte Count"=w275, "Message Out"=w276, "VISA Refnum in"=w278) -> ("error out"=w274:errorcluster, "WriteOK"=w273:bool)  [unwired: 6 in]
        n93 = call <vilib>:"Clear Errors.vi"("error in (no error)"=w274) -> ("error out"=w282:errorcluster)  [unwired: 5 in, 1 out]
        n94 = Bundle By Name(cluster=w284, "ACK"=w273) -> (w283:T10)
        n95 = call <vilib>:"Add State(s) to Queue__jki_lib_state_machine.vi"("State(s) in (\"\")"=w287) -> ("States Out"=w286:string)  [unwired: 14 in]
      }
      frame "Send Continue" {
        w298 = T5 2 items=["CMD_Eval_Mode_Entry_CC1", "CMD_Eval_Mode_Entry_CC2", "CMD_Eval_Mode_Continue", "CMD_Send_DIAG_Info", "CMD_Enable_Debug_Log ", "CMD_Disable_Debug_Log ", "CMD_Send_Log_Data"] ("Command 2")
        n96 = Unbundle By Name(w299) -> ("ComPort"=w290:refnum<visa-resource-name>)
        n97 = call "GEA2 Commands Dryer CMD.vi"("Dryer Cmd"=w298) -> ("CMD Array"=w292:u8[])  [unwired: 10 in]
        n98 = call "GEA2 Serial Generate Command.vi"("Error In"=w296, "CMD Array"=w292, "Source Destination"=w293) -> ("Error Out"=w295:errorcluster, "Byte Count"=w289:u32, "Message Out"=w291:u8[])  [unwired: 6 in]
        n99 = call "GEA2 Serial Send Command.vi"("error in (no error)"=w295, "Byte Count"=w289, "Message Out"=w291, "VISA Refnum in"=w290) -> ("error out"=w294:errorcluster, "WriteOK"=w288:bool)  [unwired: 6 in]
        n100 = local write "WriteOK"(w288) -> ()
        n101 = call "UTILITY Delay mS.vi"("Error In"=w294, "milliseconds to wait"=u32 100) -> ("Error Out"=w297:errorcluster)  [unwired: 13 in]
        n102 = call <vilib>:"Add State(s) to Queue__jki_lib_state_machine.vi"("State(s) in (\"\")"=w302) -> ("States Out"=w301:string)  [unwired: 14 in]
      }
      frame "Send En Debug Log" {
        w316 = T5 4 items=["CMD_Eval_Mode_Entry_CC1", "CMD_Eval_Mode_Entry_CC2", "CMD_Eval_Mode_Continue", "CMD_Send_DIAG_Info", "CMD_Enable_Debug_Log ", "CMD_Disable_Debug_Log ", "CMD_Send_Log_Data"] ("Command 2")
        n103 = Unbundle By Name(w317) -> ("ComPort"=w307:refnum<visa-resource-name>, "ACK"=w314:bool)
        n104 = call "GEA2 Commands Dryer CMD.vi"("Dryer Cmd"=w316) -> ("CMD Array"=w309:u8[])  [unwired: 10 in]
        n105 = call "GEA2 Serial Generate Command.vi"("Error In"=w311, "CMD Array"=w309, "Source Destination"=w310) -> ("Error Out"=w305:errorcluster, "Byte Count"=w306:u32, "Message Out"=w308:u8[])  [unwired: 6 in]
        n106 = call "GEA2 Serial Send Command.vi"("error in (no error)"=w305, "Byte Count"=w306, "Message Out"=w308, "VISA Refnum in"=w307) -> ("error out"=w303:errorcluster, "WriteOK"=w304:bool)  [unwired: 6 in]
        n107 = And(x=w314, y=w304) -> (x .and. y?=w315:bool)
        n108 = call "UTILITY Delay mS.vi"("Error In"=w303, "milliseconds to wait"=u32 500) -> ("Error Out"=w313:errorcluster)  [unwired: 13 in]
        n109 = call <vilib>:"Clear Errors.vi"("error in (no error)"=w313) -> ("error out"=w312:errorcluster)  [unwired: 5 in, 1 out]
        n110 = local write "WriteOK"(w315) -> ()
        n111 = call <vilib>:"Add State(s) to Queue__jki_lib_state_machine.vi"("State(s) in (\"\")"=w320) -> ("States Out"=w319:string)  [unwired: 14 in]
      }
      frame "Send ASCII" {
        w328 = T5 6 items=["CMD_Eval_Mode_Entry_CC1", "CMD_Eval_Mode_Entry_CC2", "CMD_Eval_Mode_Continue", "CMD_Send_DIAG_Info", "CMD_Enable_Debug_Log ", "CMD_Disable_Debug_Log ", "CMD_Send_Log_Data"] ("Command")
        n112 = Unbundle By Name(w330) -> ("ComPort"=w332:refnum<visa-resource-name>)
        n113 = call "GEA2 Commands Dryer CMD.vi"("Dryer Cmd"=w328) -> ("CMD Array"=w327:u8[])  [unwired: 10 in]
        n114 = call "GEA2 Serial Generate Command.vi"("Error In"=w331, "CMD Array"=w327, "Source Destination"=w329) -> ("Error Out"=w324:errorcluster, "Byte Count"=w325:u32, "Message Out"=w326:u8[])  [unwired: 6 in]
        n115 = call "GEA2 Serial Send Command.vi"("error in (no error)"=w324, "Byte Count"=w325, "Message Out"=w326, "VISA Refnum in"=w332) -> ("error out"=w322:errorcluster)  [unwired: 6 in, 1 out]
        n116 = call "UTILITY Delay mS.vi"("Error In"=w322, "milliseconds to wait"=u32 10) -> ("Error Out"=w321:errorcluster)  [unwired: 13 in]
        n117 = call <vilib>:"Add State(s) to Queue__jki_lib_state_machine.vi"("State(s) in (\"\")"=w334) -> ("States Out"=w333:string)  [unwired: 14 in]
      }
      frame "Send Status" {
        w337 = T5 3 items=["CMD_Eval_Mode_Entry_CC1", "CMD_Eval_Mode_Entry_CC2", "CMD_Eval_Mode_Continue", "CMD_Send_DIAG_Info", "CMD_Enable_Debug_Log ", "CMD_Disable_Debug_Log ", "CMD_Send_Log_Data"] ("Command")
        n118 = Unbundle By Name(w344) -> ("ComPort"=w342:refnum<visa-resource-name>)
        n119 = call "GEA2 Commands Dryer CMD.vi"("Dryer Cmd"=w337) -> ("CMD Array"=w336:u8[])  [unwired: 10 in]
        n120 = call "GEA2 Serial Generate Command.vi"("Error In"=w338, "CMD Array"=w336, "Source Destination"=w343) -> ("Error Out"=w339:errorcluster, "Byte Count"=w340:u32, "Message Out"=w341:u8[])  [unwired: 6 in]
        n121 = call "GEA2 Serial Send Command.vi"("error in (no error)"=w339, "Byte Count"=w340, "Message Out"=w341, "VISA Refnum in"=w342) -> ("error out"=w335:errorcluster)  [unwired: 6 in, 1 out]
        n122 = call <vilib>:"Add State(s) to Queue__jki_lib_state_machine.vi"("State(s) in (\"\")"=w346) -> ("States Out"=w345:string)  [unwired: 14 in]
      }
      frame "ReadData" {
        w350 = u32 8  # Idle Time
        (unwired) -1073807252  # Buffer Overflow
        # "Try to make sure not in mid of transmission"
        # "Read the port:"
        n123 = Unbundle By Name(w360) -> ("ComPort"=w352:refnum<visa-resource-name>)
        n124 = call "GEA2 Serial Wait for Bus Idle.vi"("Error In"=w354, "Idle Time"=w350, "ComPort"=w352) -> ("error out"=w353:errorcluster, "Bytes at Port"=w351:u32)  [unwired: 7 in]
        "Bytes At Port" <- w351
        n125 = To Long Integer(number=w351) -> (32bit integer=w348:i32)
        n126 = VISA Read(VISA resource name=w352, byte count=w351, error in (no error)=w353) -> (read buffer=w359:string, error out=w347:errorcluster)  [unwired: 2 out]
        n127 = String To Byte Array(string=w359) -> (unsigned byte array=w358:u8[])
        n128 = Bundle By Name(cluster=w360, "Total Bytes Read"=w348, "ReadArray"=w358, "CRCArray"=u8[] [] ("ReadArray"), "Current Read Index"=0) -> (w357:T10)
        n129 = Bundle By Name(cluster=w357, "Dryer Status Serial Data In.Command:Data"="") -> (w356:T10)
        n130 = call <vilib>:"Add State(s) to Queue__jki_lib_state_machine.vi"("State(s) in (\"\")"=w363) -> ("States Out"=w362:string)  [unwired: 14 in]
      }
      frame " ------- ReadData ------------ " {
        # "Template Separator\n(You can make a copy of, or modify, this frame)"
        n131 = call <vilib>:"Add State(s) to Queue__jki_lib_state_machine.vi"("State(s) in (\"\")"=w367) -> ("States Out"=w366:string)  [unwired: 14 in]
      }
      frame "Data: Parse" {
        n132 = Unbundle By Name(w370) -> ("Total Bytes Read"=w368:i32)
        n133 = To Long Integer(number=w368) -> (32bit integer=w372:i32)
        n134 = Equal To 0?(x=w372) -> (x = 0?=w371:bool)
        n135 = case shown="False" w371 {
          tunnel: ["Interpret Bytes" ("State(s) in Front (\"\")") "Parse: STX\nParse: Destination\nParse: Length\nParse: Source\nParse: Bytes Data\nParse: CRC1\nParse: CRC2\nCheckCRC\nParse: ETX\nInterpret Bytes\nCheck Complete" ("State(s) in Front (\"\")")] -> w373
          tunnel: w370 -> [w379 w381]
          tunnel: [w378 w381] -> w369
          frame True {
            n136 = Bundle By Name(cluster=w379, "Bytes Data"=u8[] []) -> (w378:T10)
          }
          frame False {
          }
        }
        n137 = call <vilib>:"Add State(s) to Queue__jki_lib_state_machine.vi"("State(s) in Front (\"\")"=w373, "State(s) in (\"\")"=w376) -> ("States Out"=w375:string)  [unwired: 13 in]
      }
      frame "Parse: STX" {
        n138 = Unbundle By Name(w394) -> ("Total Bytes Read"=w387:i32, "Current Read Index"=w388:i32, "ReadArray"=w390:u8[])
        n139 = call "GEA2 Serial Get STX.vi"("Error In"=w386, "ReadArray"=w390, "Current Read Index in"=w388, "Total Bytes Read"=w387) -> ("Error Out"=w385:errorcluster, "Complete Message"=w384:bool, "Current Read Index out"=w383:i32)  [unwired: 4 in, 1 out]
        n140 = case shown="False" w384 {
          tunnel: w385 -> [w401 w403]
          tunnel: [w399 w403] -> w392
          tunnel: ["Exit" ("State(s) in Front (\"\")") "" ("State(s) in Front (\"\")")] -> w391
          frame False {
            # "Partial Message"
            n141 = local write "Partial Message"(TRUE ("Partial Message")) -> ()
            n142 = Bundle By Name(cluster=w401, "source"="Partial GEA Message") -> (w399:errorcluster)
          }
          frame True {
          }
        }
        n143 = Bundle By Name(cluster=w394, "Current Read Index"=w383, "Bytes Data"=u8[] []) -> (w393:T10)
        n144 = call <vilib>:"Add State(s) to Queue__jki_lib_state_machine.vi"("State(s) in Front (\"\")"=w391, "State(s) in (\"\")"=w396) -> ("States Out"=w395:string)  [unwired: 13 in]
      }
      frame "Parse: Source" {
        n145 = Unbundle By Name(w413) -> ("CRCArray"=w411:u8[], "ReadArray"=w408:u8[], "Current Read Index"=w409:i32)
        n146 = call "GEA2 Serial Get Source Address.vi"("Error In"=w405, "Current Read Index"=w409, "ReadArray"=w408, "CRCArray"=w411) -> ("Error Out"=w404:errorcluster, "Source Address"=→"Source Read":u8, "Current Read Index"=w407:i32, "CRC Array"=w410:u8[])  [unwired: 4 in]
        n147 = Bundle By Name(cluster=w413, "CRCArray"=w410, "Current Read Index"=w407) -> (w412:T10)
        n148 = call <vilib>:"Add State(s) to Queue__jki_lib_state_machine.vi"("State(s) in (\"\")"=w415) -> ("States Out"=w414:string)  [unwired: 14 in]
      }
      frame "Parse: Length" {
        n149 = Unbundle By Name(w431) -> ("Total Bytes Read"=w426:i32, "ReadArray"=w421:u8[], "CRCArray"=w428:u8[], "Current Read Index"=w420:i32)
        n150 = call "GEA2 Serial Command Length.vi"("Current Read Index"=w420, "Error In"=w417, "CRCArray"=w428, "ReadArray"=w421, "Total Bytes Read"=w426) -> ("Error Out"=w416:errorcluster, "Bytes Remaining"=w419:u8, "CRC Array"=w429:u8[], "Current Read Index"=w425:i32, "Boolean"=w427:bool, "Length"=→"Length":u8)  [unwired: 1 in]
        "Partial Message" <- w427
        n151 = Bundle By Name(cluster=w431, "Current Read Index"=w425, "CRCArray"=w429, "Bytes Remaining"=w419) -> (w430:T10)
        n152 = local read "Mode"() -> (w424:T6)
        n153 = case shown="True" w427 {
          tunnel: w424 -> [_ w435]
          tunnel: [w433 w434] -> w422
          tunnel: w423 -> [w433 _]
          frame False {
          }
          frame True {
            n154 = case shown="\"Read Continuous\"" w435 {
              tunnel: ["Exit" ("State(s) in Front (\"\")") "Read Continue" ("State(s) in Front (\"\")")] -> w434
              frame "Init Com Port", Default {
              }
              frame "Read Continuous" {
              }
            }
          }
        }
        n155 = call <vilib>:"Add State(s) to Queue__jki_lib_state_machine.vi"("State(s) in (\"\")"=w422) -> ("States Out"=w432:string)  [unwired: 14 in]
      }
      frame "Parse: Destination" {
        n156 = Unbundle By Name(w447) -> ("ReadArray"=w442:u8[], "Current Read Index"=w444:i32)
        n157 = call "GEA2 Serial Get Destination Address.vi"("Error In"=w439, "Source Destination"=w441, "Current Read Index"=w444, "ReadArray"=w442) -> ("Error Out"=w438:errorcluster, "Destination Read"=→"Destination Read":u8, "CRC Array"=w443:u8[], "Current Read Index"=w445:i32)  [unwired: 3 in, 1 out]
        n158 = Bundle By Name(cluster=w447, "Current Read Index"=w445, "CRCArray"=w443) -> (w446:T10)
        n159 = call <vilib>:"Add State(s) to Queue__jki_lib_state_machine.vi"("State(s) in (\"\")"=w449) -> ("States Out"=w448:string)  [unwired: 14 in]
      }
      frame "Parse: Bytes Data" {
        n160 = Unbundle By Name(w464) -> ("Current Read Index"=w450:i32, "ReadArray"=w453:u8[], "CRCArray"=w461:u8[], "Bytes Remaining"=w460:u8, "Bytes Data"=w458:u8[])
        n161 = call "GEA2 Serial Get Bytes Data.vi"("Bytes Data"=w458, "Current Read Index"=w450, "Error In"=w452, "Bytes Remaining"=w460, "CRCArray"=w461, "ReadArray"=w453) -> ("Error Out"=w451:errorcluster, "Bytes Remaining"=w454:u8, "CRC Array"=w462:u8[], "Current Read Index"=w459:i32, "Bytes Data Out"=w457:u8[], "Parse Bytes"=w456:bool)
        n162 = Bundle By Name(cluster=w464, "Current Read Index"=w459, "CRCArray"=w462, "Bytes Remaining"=w454, "Bytes Data"=w457) -> (w463:T10)
        n163 = case shown="True" w456 {
          tunnel: ["" ("State(s) in Front (\"\")") "Parse: Bytes Data" ("State(s) in Front (\"\")")] -> w455
          frame False {
          }
          frame True {
          }
        }
        n164 = call <vilib>:"Add State(s) to Queue__jki_lib_state_machine.vi"("State(s) in Front (\"\")"=w455, "State(s) in (\"\")"=w466) -> ("States Out"=w465:string)  [unwired: 13 in]
      }
      frame "Parse: CRC1" {
        n165 = Unbundle By Name(w476) -> ("ReadArray"=w473:u8[], "Current Read Index"=w472:i32)
        n166 = call "GEA2 Serial Get CRC1.vi"("Error In"=w470, "Current Read Index"=w472, "ReadArray"=w473) -> ("Error Out"=w469:errorcluster, "CRC Read"=w471:u8[], "Current Read Index"=w474:i32)  [unwired: 6 in]
        n167 = Bundle By Name(cluster=w476, "Current Read Index"=w474, "CRCRead"=w471) -> (w475:T10)
        n168 = call <vilib>:"Add State(s) to Queue__jki_lib_state_machine.vi"("State(s) in (\"\")"=w478) -> ("States Out"=w477:string)  [unwired: 14 in]
      }
      frame "Parse: CRC2" {
        n169 = Unbundle By Name(w487) -> ("ReadArray"=w481:u8[], "CRCRead"=w483:u8[], "Current Read Index"=w482:i32)
        n170 = call "GEA2 Serial Get CRC2.vi"("Error In"=w480, "Current Read Index"=w482, "CRCRead"=w483, "ReadArray"=w481) -> ("Error Out"=w479:errorcluster, "CRC Read"=w484:u8[], "Current Read Index"=w485:i32)  [unwired: 5 in]
        n171 = Bundle By Name(cluster=w487, "Current Read Index"=w485, "CRCRead"=w484) -> (w486:T10)
        n172 = call <vilib>:"Add State(s) to Queue__jki_lib_state_machine.vi"("State(s) in (\"\")"=w489) -> ("States Out"=w488:string)  [unwired: 14 in]
      }
      frame "CheckCRC" {
        n173 = Unbundle By Name(w494) -> ("CRCRead"=w491:u8[], "CRCArray"=w495:u8[])
        n174 = call "GEA2 Serial Check CRC.vi"("error in (no error)"=w496, "CRCArray"=w495, "CRCRead in"=w491) -> ("error out"=w492:errorcluster, "CRC Match"=w490:bool)  [unwired: 7 in]
        "CRC Match" <- w490
        n175 = Bundle By Name(cluster=w494, "CRC"=w490) -> (w493:T10)
        n176 = call <vilib>:"Add State(s) to Queue__jki_lib_state_machine.vi"("State(s) in (\"\")"=w498) -> ("States Out"=w497:string)  [unwired: 14 in]
      }
      frame "Parse: ETX" {
        n177 = Unbundle By Name(w508) -> ("ReadArray"=w503:u8[], "Current Read Index"=w501:i32)
        n178 = call "GEA2 Serial Get ETX.vi"("Error In"=w500, "Current Read Index"=w501, "ReadArray"=w503) -> ("Error Out"=w499:errorcluster, "ETX = E3"=w506:bool, "Current Read Index"=w502:i32)  [unwired: 6 in]
        n179 = Bundle By Name(cluster=w508, "Current Read Index"=w502) -> (w507:T10)
        n180 = case shown="False" w506 {
          tunnel: w499 -> [w514 w517]
          tunnel: [w511 w517] -> w505
          tunnel: ["Exit" ("State(s) in Front (\"\")") "" ("State(s) in Front (\"\")")] -> w504
          frame False {
            n181 = call "GEA2 Serial Error Bool Enumerator.vi"("Error Enum"=GEA2_Serial_Dryer_Error_Enumeration."GEA2 ETX", "Error In"=w514, "Error?"=TRUE) -> ("Error Out"=w511:errorcluster)  [unwired: 6 in]
          }
          frame True {
          }
        }
        n182 = call <vilib>:"Add State(s) to Queue__jki_lib_state_machine.vi"("State(s) in Front (\"\")"=w504, "State(s) in (\"\")"=w510) -> ("States Out"=w509:string)  [unwired: 13 in]
      }
      frame "SendACK" {
        n183 = Unbundle By Name(w519) -> ("ComPort"=w521:refnum<visa-resource-name>, "CRC"=w518:bool)
        n184 = call "GEA2 Serial Send ACK.vi"("error in (no error)"=w522, "CRC"=w518, "VISA Refnum in"=w521) -> ("error out"=w520:errorcluster)  [unwired: 8 in]
        n185 = call <vilib>:"Add State(s) to Queue__jki_lib_state_machine.vi"("State(s) in (\"\")"=w524) -> ("States Out"=w523:string)  [unwired: 14 in]
      }
      frame "Interpret Bytes" {
        n186 = Unbundle By Name(w529) -> ("Bytes Data"=w531:u8[], "ComPort"=w525:refnum<visa-resource-name>, "Dryer Status Serial Data In"=w530:T2)
        "DataReturned" <- w531
        n187 = call "GEA2 Serial Dryer Status.vi"("Bytes Comm"=w531, "VISA resource name"=w525, "Dryer Status Serial Data In"=w530) -> ("Dryer Status Serial Data Out"=w526:T2)  [unwired: 12 in]
        "Dryer Status Serial Data Out" <- w526
        n188 = Unbundle By Name(w526) -> ("Command:Data"=→"Com:Data":string)
        n189 = Bundle By Name(cluster=w529, "Dryer Status Serial Data In"=w526) -> (w528:T10)
        n190 = call <vilib>:"Add State(s) to Queue__jki_lib_state_machine.vi"("State(s) in (\"\")"=w534) -> ("States Out"=w533:string)  [unwired: 14 in]
      }
      frame "Check Complete" {
        n191 = Unbundle By Name(w537) -> ("Total Bytes Read"=w541:i32, "Current Read Index"=w540:i32, "Reset MSG Count"=w538:bool)
        n192 = Subtract(x=w541, y=w540) -> (x-y=w539:i32)
        n193 = call "UTILITY Counter.vi"("Reset"=w538) -> ("Count"=→"Num Messages":dbl)  [unwired: 10 in]
        n194 = Greater?(x=w539, y=7) -> (0:w544:bool)
        n195 = case shown="True" w544 {
          tunnel: [_ "Parse: STX\nParse: Destination\nParse: Length\nParse: Source\nParse: Bytes Data\nParse: CRC1\nParse: CRC2\nCheckCRC\nParse: ETX\nInterpret Bytes\nCheck Complete" ("State(s) in Front (\"\")")] -> w543
          frame False {
          }
          frame True {
          }
        }
        n196 = Bundle By Name(cluster=w537, "Reset MSG Count"=FALSE) -> (w536:T10)
        n197 = call <vilib>:"Add State(s) to Queue__jki_lib_state_machine.vi"("State(s) in Front (\"\")"=w543, "State(s) in (\"\")"=w548) -> ("States Out"=w547:string)  [unwired: 13 in]
      }
      frame "Read Continue" {
        n198 = local read "Com:Data"() -> (w567:string)
        n199 = local read "Bytes At Port"() -> (w562:u32)
        n200 = Unbundle By Name(w555) -> ("Reset Pulse"=w554:bool)
        n201 = Search and Replace String(input string=w567, search string="No Com", replace string="" ("replace string (\"\")")) -> (result string=w564:string)  [unwired: 5 in, 3 out]
        n202 = To Long Integer(number=w562) -> (32bit integer=w558:i32)
        n203 = To Long Integer(number=u32 7 ("y")) -> (32bit integer=w557:i32)
        n204 = call <vilib>:"Trim Whitespace.vi"("string"=w564) -> ("trimmed string"=w563:string)  [unwired: 1 in]
        n205 = Subtract(x=w558, y=w557) -> (x-y=w560:i32)
        n206 = Greater Than 0?(x=w560) -> (x > 0?=w559:bool)
        n207 = call "UTILITY Counter.vi"("Reset"=w554) -> ("Count"=→"Read Pulse":dbl)  [unwired: 10 in]
        n208 = case shown="True" w559 {
          tunnel: w563 -> [_ w582]
          tunnel: [w578 w579] -> w569
          frame False {
            n209 = local read "Com:Data Buffer"() -> (w578:string)
          }
          frame True {
            n210 = local read "Com:Data Buffer"() -> (w580:string)
            n211 = Concatenate Strings(w582, "\n", w580) -> (w579:string)
            n212 = local write "Com:Data Buffer"(w579) -> ()
          }
        }
        n213 = flat-sequence {
          tunnel: ["ReadData\nData: Parse\nRead Continue"] -> w552
          tunnel: w569 -> [w576]
          frame #0 {
            n214 = local write "Com:Data"(w576) -> ()
            n215 = Wait (ms)(milliseconds to wait=u32 2000) -> ()  [unwired: 1 out]
          }
        }
        n216 = Bundle By Name(cluster=w555, "Reset Pulse"=FALSE ("Reset MSG Count"), "Dryer Status Serial Data In.Command:Data"="") -> (w571:T10)
        n217 = local read "Exit"() -> (w553:bool)
        n218 = Select(t="Exit", s=w553, f=w552) -> (s? t:f=w550:string)
        n219 = call <vilib>:"Add State(s) to Queue__jki_lib_state_machine.vi"("State(s) in Front (\"\")"=w550, "State(s) in (\"\")"=w574) -> ("States Out"=w573:string)  [unwired: 13 in]
      }
    }
    n220 = case shown="True" "Debug" {
      tunnel: w33 -> [w43 w46]
      tunnel: w32 -> [_ w45]
      tunnel: [w43 w44] -> w31
      frame False {
      }
      frame True {
        n221 = Build Array (concatenate)(w46, w45) -> (w44:string[])
        "State Array" <- w44
      }
    }
    n222 = local write "Error Out"(w34) -> ()
  }
  n223 = disable-structure shown="Disabled" {
    frame Disabled {
      # "Work on this...it will make nicer"
      n224 = call "GEA2 Serial Get STX.vi"() -> ("Error Out"=w606:errorcluster, "Current Read Index out"=w598:i32, "Read Array Out"=w584:u8[])  [unwired: 8 in, 1 out]
      n225 = call "GEA2 Serial Get Destination Address.vi"("Error In"=w606, "Source Destination"="Source Destination 2", "Current Read Index"=w598, "ReadArray"=w584) -> ("Error Out"=w605:errorcluster, "CRC Array"=w597:u8[], "Current Read Index"=w596:i32)  [unwired: 3 in, 2 out]
      n226 = call "GEA2 Serial Command Length.vi"("Current Read Index"=w596, "Error In"=w605, "CRCArray"=w597, "ReadArray"=w584, "Total Bytes Read"="Total Bytes Read") -> ("Error Out"=w604:errorcluster, "Bytes Remaining"=w590:u8, "CRC Array"=w593:u8[], "Current Read Index"=w594:i32)  [unwired: 1 in, 2 out]
      n227 = call "GEA2 Serial Get Source Address.vi"("Error In"=w604, "Current Read Index"=w594, "ReadArray"=w584, "CRCArray"=w593) -> ("Error Out"=w603:errorcluster, "Current Read Index"=w591:i32, "CRC Array"=w592:u8[])  [unwired: 4 in, 1 out]
      n228 = while {
        tunnel: w592 -> [w616]
        tunnel: w591 -> [w615]
        tunnel: w584 -> [w614]
        shift-right: [w617] -> w602
        shift-left: w603 -> [w618]
        tunnel: w590 -> [w613]
        shift-right: [w611] -> _
        shift-left: u8[] [] ("Bytes Data") -> [w612]
        tunnel: [w610] -> w588
        tunnel: [w607] -> _
        stop <- w609 stop-if-true
        n229 = call "GEA2 Serial Get Bytes Data.vi"("Bytes Data"=w612, "Current Read Index"=w615, "Error In"=w618, "Bytes Remaining"=w613, "CRCArray"=w616, "ReadArray"=w614) -> ("Error Out"=w617:errorcluster, "CRC Array"=w607:u8[], "Current Read Index"=w610:i32, "Bytes Data Out"=w611:u8[], "Parse Bytes"=w608:bool)  [unwired: 1 out]
        n230 = Not(x=w608) -> (.not. x?=w609:bool)
      }
      n231 = call "GEA2 Serial Get CRC1.vi"("Error In"=w602, "Current Read Index"=w588, "ReadArray"=w584) -> ("Error Out"=w601:errorcluster, "CRC Read"=w586:u8[], "Current Read Index"=w587:i32)  [unwired: 6 in]
      n232 = call "GEA2 Serial Get CRC2.vi"("Error In"=w601, "Current Read Index"=w587, "CRCRead"=w586, "ReadArray"=w584) -> ("Error Out"=w600:errorcluster, "CRC Read"=w585:u8[])  [unwired: 5 in, 1 out]
      n233 = call "GEA2 Serial Check CRC.vi"("error in (no error)"=w600, "CRCArray"=w585) -> ("error out"=w599:errorcluster)  [unwired: 8 in, 1 out]
      n234 = call "GEA2 Serial Get ETX.vi"("Error In"=w599, "ReadArray"=w584) -> ()  [unwired: 7 in, 3 out]
    }
    frame Enabled {
    }
  }
  n235 = Unbundle By Name(w6) -> ("Error Out Flag"=w5:bool)
  n236 = Bundle By Name(cluster=w9, "status"=w5) -> (→"Error Out":errorcluster)
